vi "Test Combinations of Broken Wells_Memo.vi"(10 "broken streaks":u8[](array[numeric]), 11 "map":i8[](array[numeric])) -> (3 "possible combinations":u64)   [LabVIEW 2022 SP3]
uses:
  <vilib>/Utility/miscctls.llb/LVMapReplaceAction.ctl
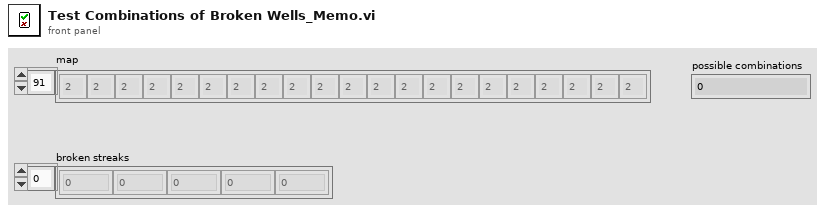
[diagram p1: front panel]
types:
  T1 = typedef "LVMapReplaceAction.ctl" = enum32{"Modify Entry only if found", "Add or Modify Entry", "Delete Entry"}
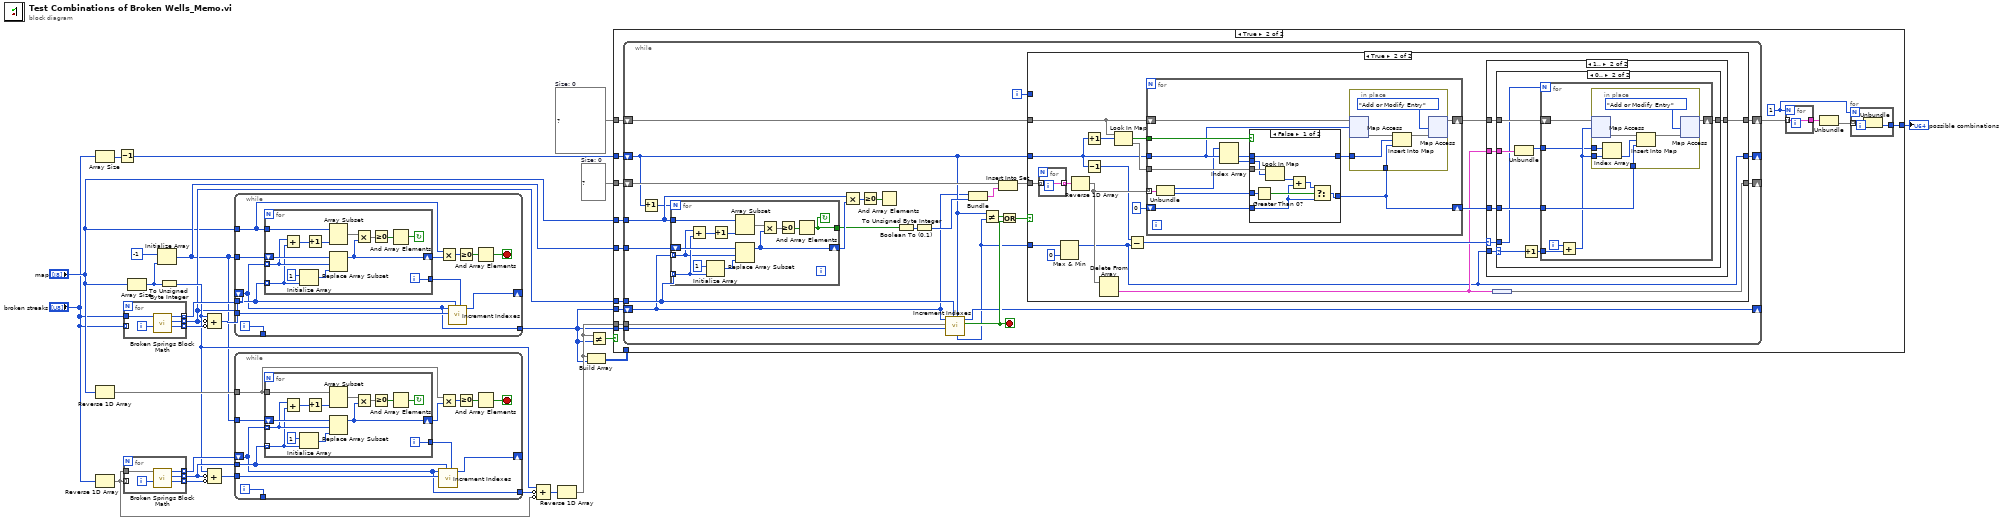
[diagram p0: block diagram]
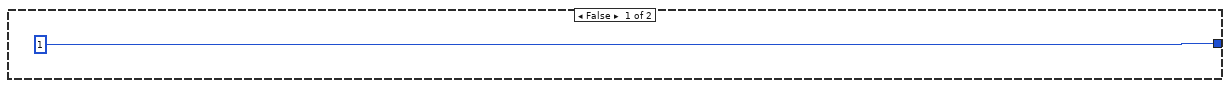
[diagram p2: hidden frame]
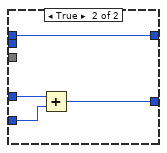
[diagram p6: hidden frame]
diagram:
  w6 = set{cluster{u8[], u8}} {}  # Size: 0
  w10 = map{i32, map{u8, u64}} {}  # Size: 0
  n1 = Array Size(array="broken streaks") -> (size(s)=w3:i32)
  n2 = Reverse 1D Array(array="map") -> (reversed array=w23:i8[])
  n3 = Reverse 1D Array(array="broken streaks") -> (reversed array=w17:u8[])
  n4 = Decrement(x=w3) -> (x-1=w2:i32)
  n5 = for {
    tunnel: "broken streaks" -> [w32]
    tunnel: "broken streaks" -> [_] mode=indexing
    tunnel: [w30] -> w26 mode=indexing
    tunnel: [w29] -> w12 mode=indexing
    tunnel: [w28] -> w27 mode=indexing
    i -> [w31]
    n6 = call "Broken Springs Block Math.vi"("index"=w31, "contiguous length of broken springs"=w32) -> ("right total"=w28:u8, "current index broken streak length"=w29:u8, "left total"=w30:u8)  [unwired: 7 in]
  }
  n7 = for {
    tunnel: w17 -> [w37]
    tunnel: w17 -> [_] mode=indexing
    tunnel: [w35] -> w21 mode=indexing
    tunnel: [w34] -> w20 mode=indexing
    tunnel: [w33] -> w22 mode=indexing
    i -> [w36]
    n8 = call "Broken Springs Block Math.vi"("index"=w36, "contiguous length of broken springs"=w37) -> ("right total"=w33:u8, "current index broken streak length"=w34:u8, "left total"=w35:u8)  [unwired: 7 in]
  }
  n9 = Array Size(array="map") -> (size(s)=w24:i32)
  n10 = Initialize Array(i8 -1 ("unsigned 8bit integer"), w24) -> (w11:i8[])
  n11 = To Unsigned Byte Integer(number=w24) -> (unsigned 8bit integer=w15:u8)
  n12 = Compound Arithmetic op=ADD(w15, invert w12, invert w27) -> (w14:u8[])
  n13 = Compound Arithmetic op=ADD(w15, invert w20, invert w22) -> (w19:u8[])
  n14 = while {
    tunnel: w11 -> [w49]
    tunnel: w12 -> [w46]
    shift-right: [w47] -> _
    shift-left: w26 -> [w43]
    tunnel: w14 -> [w48]
    tunnel: "map" -> [w38]
    tunnel: [w44] -> _
    tunnel: [w43] -> w1
    i -> [w44]
    stop <- w39 stop-if-true
    n15 = for {
      tunnel: w46 -> [w58] mode=indexing
      shift-right: [w55] -> w40
      shift-left: w49 -> [w63]
      tunnel: w43 -> [w59] mode=indexing
      tunnel: w38 -> [w60]
      tunnel: [w53] -> w45
      i -> [w53]
      stop <- w51 continue-if-true
      n16 = Add(x=w59, y=w58) -> (x+y=w57:u8)
      n17 = Initialize Array(i8 1 ("unsigned 8bit integer"), w58) -> (w62:i8[])
      n18 = Increment(x=w57) -> (x+1=w50:u8)
      n19 = Array Subset(array=w60, length=w50) -> (w56:i8[])  [unwired: 1 in]
      n20 = Replace Array Subset(array=w63, new element=w62, index=w59) -> (w55:i8[])
      n21 = Multiply(x=w56, y=w55) -> (x*y=w52:i8[])
      n22 = Greater Or Equal To 0?(x=w52) -> (x >= 0?=w54:bool[])
      n23 = And Array Elements(Boolean array=w54) -> (logical AND=w51:bool)
    }
    n24 = Multiply(x=w38, y=w40) -> (x*y=w41:i8[])
    n25 = call "Increment Indexes.vi"("group index to increment"=w45, "lengths"=w46, "max indexes"=w48, "previous indexes"=w43) -> ("next indexes"=w47:u8[])  [unwired: 5 in, 2 out]
    n26 = Greater Or Equal To 0?(x=w41) -> (x >= 0?=w42:bool[])
    n27 = And Array Elements(Boolean array=w42) -> (logical AND=w39:bool)
  }
  n28 = while {
    tunnel: w11 -> [w75]
    tunnel: w20 -> [w72]
    shift-right: [w73] -> _
    shift-left: w21 -> [w69]
    tunnel: w19 -> [w74]
    tunnel: w23 -> [w64]
    tunnel: [w70] -> _
    tunnel: [w69] -> w18
    i -> [w70]
    stop <- w66 stop-if-true
    n29 = for {
      tunnel: w72 -> [w84] mode=indexing
      shift-right: [w81] -> w65
      shift-left: w75 -> [w89]
      tunnel: w69 -> [w85] mode=indexing
      tunnel: w64 -> [w86]
      tunnel: [w79] -> w71
      i -> [w79]
      stop <- w77 continue-if-true
      n30 = Add(x=w85, y=w84) -> (x+y=w83:u8)
      n31 = Initialize Array(i8 1 ("unsigned 8bit integer"), w84) -> (w88:i8[])
      n32 = Increment(x=w83) -> (x+1=w76:u8)
      n33 = Array Subset(array=w86, length=w76) -> (w82:i8[])  [unwired: 1 in]
      n34 = Replace Array Subset(array=w89, new element=w88, index=w85) -> (w81:i8[])
      n35 = Multiply(x=w82, y=w81) -> (x*y=w78:i8[])
      n36 = Greater Or Equal To 0?(x=w78) -> (x >= 0?=w80:bool[])
      n37 = And Array Elements(Boolean array=w80) -> (logical AND=w77:bool)
    }
    n38 = call "Increment Indexes.vi"("group index to increment"=w71, "lengths"=w72, "max indexes"=w74, "previous indexes"=w69) -> ("next indexes"=w73:u8[])  [unwired: 5 in, 2 out]
    n39 = Multiply(x=w64, y=w65) -> (x*y=w68:i8[])
    n40 = Greater Or Equal To 0?(x=w68) -> (x >= 0?=w67:bool[])
    n41 = And Array Elements(Boolean array=w67) -> (logical AND=w66:bool)
  }
  n42 = Compound Arithmetic op=ADD(w15, invert w18, invert w17) -> (w16:u8[])
  n43 = Reverse 1D Array(array=w16) -> (reversed array=w13:u8[])
  n44 = Build Array(w13, w1) -> (w8:u8[][])
  n45 = Not Equal?(x=w13, y=w1) -> (x != y?=w9:bool)
  n46 = case shown="True" w9 {
    tunnel: "map" -> [_ w104]
    tunnel: w1 -> [_ w103]
    tunnel: w13 -> [_ w102]
    tunnel: w12 -> [_ w101]
    tunnel: w11 -> [_ w100]
    tunnel: w6 -> [_ w99]
    tunnel: w10 -> [_ w98]
    tunnel: w8 -> [_ _]
    tunnel: [u64 1 ("possible combinations") w91] -> w7
    tunnel: w2 -> [_ w94]
    tunnel: w1 -> [_ w93]
    frame False {
    }
    frame True {
      w92 = 1
      n47 = while {
        tunnel: w100 -> [w131]
        tunnel: w101 -> [w120]
        shift-right: [w113] -> _
        shift-left: w103 -> [w106]
        tunnel: w102 -> [w119]
        tunnel: w104 -> [w127]
        shift-right: [w122] -> _
        shift-left: w99 -> [w126]
        shift-right: [w117] -> w97
        shift-left: w98 -> [w118]
        shift-right: [w116] -> _
        shift-left: w94 -> [w109]
        tunnel: w93 -> [w107]
        i -> [w112]
        stop <- w124 stop-if-true
        n48 = Increment(x=w109) -> (x+1=w110:i32)
        n49 = for {
          N: w110 -> [_]
          tunnel: w120 -> [w133] mode=indexing
          shift-right: [w138] -> w128
          shift-left: w131 -> [w144]
          tunnel: w106 -> [w132] mode=indexing
          tunnel: w127 -> [w141]
          tunnel: [w134] -> w108
          stop <- w134 continue-if-true
          n50 = Add(x=w132, y=w133) -> (x+y=w140:u8)
          n51 = Initialize Array(i8 1 ("unsigned 8bit integer"), w133) -> (w143:i8[])
          n52 = Increment(x=w140) -> (x+1=w135:u8)
          n53 = Array Subset(array=w141, length=w135) -> (w139:i8[])  [unwired: 1 in]
          n54 = Replace Array Subset(array=w144, new element=w143, index=w132) -> (w138:i8[])
          n55 = Multiply(x=w139, y=w138) -> (x*y=w136:i8[])
          n56 = Greater Or Equal To 0?(x=w136) -> (x >= 0?=w137:bool[])
          n57 = And Array Elements(Boolean array=w137) -> (logical AND=w134:bool)
        }
        n58 = Multiply(x=w127, y=w128) -> (x*y=w129:i8[])
        n59 = Greater Or Equal To 0?(x=w129) -> (x >= 0?=w130:bool[])
        n60 = And Array Elements(Boolean array=w130) -> ()  [unwired: 1 out]
        n61 = Boolean To (0,1)(Boolean=w108) -> (0, 1=w114:i16)
        n62 = To Unsigned Byte Integer(number=w114) -> (unsigned 8bit integer=w111:u8)
        n63 = call "Increment Indexes.vi"("group index to increment"=w109, "lengths"=w120, "min indexes"=w107, "max indexes"=w119, "previous indexes"=w106) -> ("complete"=w124:bool, "next indexes"=w113:u8[], "actual index incremented"=w105:i32)  [unwired: 4 in]
        n64 = Bundle(w106, w111) -> (w115:cluster{u8[], u8})  [unwired: 1 in]
        n65 = Not Equal?(x=w109, y=w105) -> (x != y?=w125:bool)
        n66 = Insert Into Set(10:w115, 11:w126) -> (3:w121:set{cluster{u8[], u8}})  [unwired: 1 out]
        n67 = Or(x=w125, y=w124) -> (x .or. y?=w123:bool)
        n68 = case shown="True" w123 {
          tunnel: [w147 w157] -> w122
          tunnel: w121 -> [w147 w166]
          tunnel: w118 -> [w146 w163]
          tunnel: [w146 w154] -> w117
          tunnel: w109 -> [w145 w160]
          tunnel: [w145 w148] -> w116
          tunnel: w112 -> [_ _]
          tunnel: w105 -> [_ w150]
          frame False {
          }
          frame True {
            n69 = for {
              tunnel: w166 -> [w197] mode=indexing
              tunnel: [w197] -> w165 mode=indexing
            }
            n70 = Max & Min(x=w150, y=0) -> (max(x,y)=w148:i32)  [unwired: 1 out]
            n71 = Reverse 1D Array(array=w165) -> (reversed array=w158:cluster{u8[], u8}[])
            n72 = Increment(x=w160) -> (x+1=w159:i32)
            n73 = Decrement(x=w160) -> (x-1=w156:i32)
            n74 = Delete From Array(array=w158) -> (deleted portion=w151:cluster{u8[], u8})  [unwired: 2 in, 1 out]
            n75 = Look In Map(map=w163, key=w159) -> (key not found?=w161:bool, value=w162:map{u8, u64})  [unwired: 1 in]
            n76 = Subtract(x=w156, y=w148) -> (x-y=w155:i32)
            n77 = for {
              tunnel: w158 -> [w207] mode=indexing
              shift-right: [w208] -> w153
              shift-left: w163 -> [w200]
              tunnel: w160 -> [w201]
              shift-right: [w209] -> w152
              shift-left: u64 0 -> [w210]
              tunnel: w162 -> [w204]
              tunnel: w161 -> [w205]
              n78 = Unbundle(w207) -> (w199:u8[], w198:u8)
              n79 = Index Array(array=w199, index #1=w201) -> (element #1=w203:u8, element #2=w202:u8)  [unwired: 1 in]
              n80 = case shown="False" w205 {
                tunnel: w210 -> [w212 w223]
                tunnel: [w215 w222] -> w209
                tunnel: [w217 w220] -> w206
                tunnel: w198 -> [w216 w221]
                tunnel: w204 -> [w219 _]
                tunnel: w203 -> [w217 w220]
                tunnel: w202 -> [w218 _]
                frame False {
                  n81 = Greater Than 0?(x=w216) -> (x > 0?=w214:bool)
                  n82 = Look In Map(map=w219, key=w218) -> (value=w213:u64)  [unwired: 1 in, 1 out]
                  n83 = Add(x=w213, y=w212) -> (x+y=w211:u64)
                  n84 = Select(t=w211, s=w214, f=w212) -> (s? t:f=w215:u64)
                }
                frame True {
                  n85 = Add(x=w221, y=w223) -> (x+y=w222:u64)
                }
              }
              n86 = in-place {
                in-place-border: w209 -> [w228]
                in-place-border: w206 -> [w224]
                n87 = in-place-map #1(w200, w201) -> (w226:map{u8, u64})  [unwired: 1 in, 1 out]
                n88 = Insert Into Map(map in=w226, key=w224, value=w228) -> (map out=w225:map{u8, u64})  [unwired: 2 out]
                n89 = in-place-map #1(w225, LVMapReplaceAction."Add or Modify Entry" ("action")) -> (w208:map{i32, map{u8, u64}})  [unwired: 2 out]
              }
            }
            n90 = case shown="1.." w155 {
              selector: w155 -> [_ w168]
              tunnel: [w167 w172] -> w154
              tunnel: w153 -> [w167 w173]
              tunnel: w148 -> [_ w171]
              tunnel: w152 -> [_ w170]
              tunnel: w151 -> [_ w169]
              frame Default {
              }
              frame 1.. {
                n91 = case shown="0.." w171 {
                  selector: w171 -> [_ w180]
                  tunnel: w173 -> [w174 w182]
                  tunnel: [w174 w181] -> w172
                  tunnel: w170 -> [_ w178]
                  tunnel: w169 -> [_ w177]
                  tunnel: w168 -> [_ w175]
                  frame Default {
                  }
                  frame 0.. {
                    n92 = Unbundle(w177) -> (w176:u8[])  [unwired: 1 out]
                    n93 = Increment(x=w180) -> (x+1=w179:i32)
                    n94 = for {
                      N: w175 -> [_]
                      shift-right: [w183] -> w181
                      shift-left: w182 -> [w187]
                      tunnel: w179 -> [w189]
                      tunnel: w178 -> [w186]
                      tunnel: w176 -> [w184]
                      i -> [w188]
                      n95 = Add(x=w188, y=w189) -> (x+y=w185:i32)
                      n96 = in-place {
                        in-place-border: w186 -> [w194]
                        in-place-border: w185 -> [w193]
                        in-place-border: w184 -> [w192]
                        n97 = in-place-map #2(w187, w185) -> (w195:map{u8, u64})  [unwired: 1 in, 1 out]
                        n98 = Index Array(array=w192, index=w193) -> (element=w191:u8)
                        n99 = Insert Into Map(map in=w195, key=w191, value=w194) -> (map out=w190:map{u8, u64})  [unwired: 2 out]
                        n100 = in-place-map #2(w190, LVMapReplaceAction."Add or Modify Entry" ("action")) -> (w183:map{i32, map{u8, u64}})  [unwired: 2 out]
                      }
                    }
                  }
                }
              }
            }
            n101 = node(w151) -> (w157:set{cluster{u8[], u8}})
          }
        }
      }
      n102 = for {
        N: w92 -> [_]
        tunnel: w97 -> [w229] mode=indexing
        tunnel: [w229] -> w96
      }
      n103 = Unbundle(w96) -> (w95:map{u8, u64})  [unwired: 1 out]
      n104 = for {
        N: w92 -> [_]
        tunnel: w95 -> [w231] mode=indexing
        tunnel: [w230] -> w91
        n105 = Unbundle(w231) -> (w230:u64)  [unwired: 1 out]
      }
    }
  }
  "possible combinations" <- w7
